vi "4Pi Capture Acq Setting AE.vi"(2 "Action":T1, 7 "Acq Setting in":T2[](array[typedef])) -> (8 "Acq Setting out":T2[](array[typedef]))   [LabVIEW 2021]
uses:
  4Pi Capture Manager Controls/4Pi Capture Acq Settings.ctl
  4Pi Dual DM Control/4Pi Dual DM - Controls/4Pi Dual DM - Standard Action.ctl
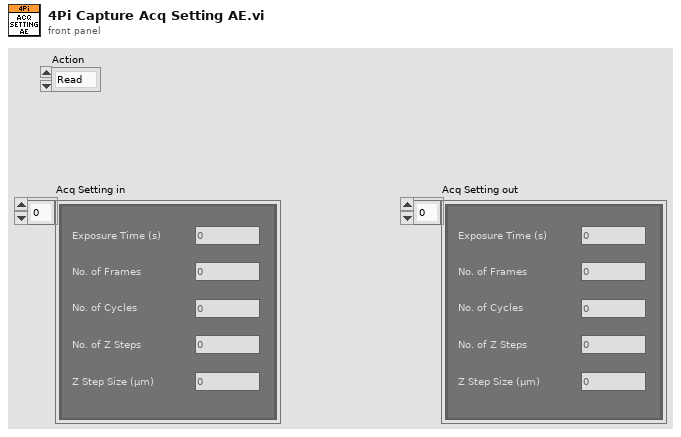
[diagram p1: front panel]
types:
  T1 = typedef "4Pi Dual DM - Standard Action.ctl" = enum16{"Read", "Write"}
  T2 = typedef "4Pi Capture Acq Settings.ctl" = cluster{"Exposure Time (s)":dbl, "No. of Frames":u32, "No. of Z Steps":u16, "No. of Cycles":u16, "Z Step Size (µm)":dbl}
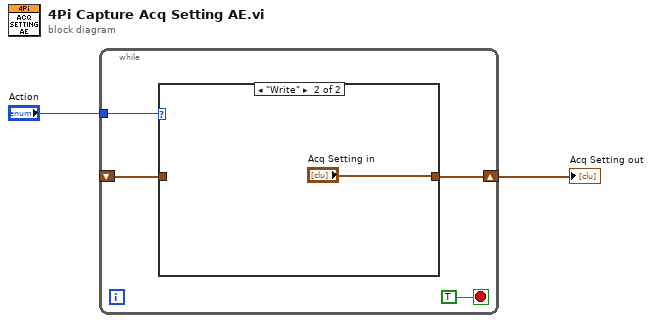
[diagram p0: block diagram]
diagram:
  n1 = while {
    tunnel: "Action" -> [w6]
    shift-right: [w5] -> w1
    shift-left: _ -> [w4]
    stop <- TRUE stop-if-true
    n2 = case shown="\"Write\"" w6 {
      tunnel: [w7 "Acq Setting in"] -> w5
      tunnel: w4 -> [w7 _]
      frame "Read", Default {
      }
      frame "Write" {
      }
    }
  }
  "Acq Setting out" <- w1
